vi "Main.vi"(11 "Module Admin":refnum<class "Delacor_lib_QMH_Module Admin.lvclass">) -> ()   [LabVIEW 2022 SP3, in "Settings.lvlib"]
doc: "This template is based off of the Queued Message Handler design pattern and the Queued Message Handler project template that ships with LabVIEW.\n\nThe main difference is that the queue is private to this module and communication between modules is performed via Broadcast and Request events.\n\nRequest events are wrapped in public API methods and are handled in the Event Handling Loop (EHL) of this VI. Any module can register for Broadcast events sent by this module. The EHL generates messages based on user interface actions.\n\nThe Message Handling Loop (MHL) processes messages generated by the EHL, or by other messages. The messages are string values, so new messages can be added easily to the Message Cases case structure in the MHL. Each message cluster can also provide an optional value for Message Data, which is a variant that can be converted to whatever message-specific data is required.\n_____\nBased on DQMH Project Template 7.0.0.1280."
uses:
  Settings.lvlib
  <vilib>/Delacor/Delacor QMH/Libraries/Module Admin_class/Delacor_lib_QMH_Module Admin.lvclass
  Module Data--cluster.ctl
  Do Something Argument--cluster.ctl
  <vilib>/Delacor/Delacor QMH/Libraries/Message Queue_class/Delacor_lib_QMH_Message Queue.lvclass/Delacor_lib_QMH_Message Queue.ctl
  Do Something Else Argument--cluster.ctl
  Do Something Else and Wait for Reply Argument--cluster.ctl
  Do Something Else and Wait (Reply Payload)--cluster.ctl
  Stop Argument--cluster.ctl
  <vilib>/Delacor/Delacor QMH/Libraries/Module Admin_class/Delacor_lib_QMH_Module Admin.lvclass/Delacor_lib_QMH_Module Admin.ctl
  Prepare Argument--cluster.ctl
  Configure Argument--cluster.ctl
  Request UI Display Argument--cluster.ctl
  Framework/UI Manager/Module Display Scenarios.ctl
  Request UI Display (Reply Payload)--cluster.ctl
  <vilib>/Utility/miscctls.llb/LVPointTypeDef.ctl
  <vilib>/Delacor/Delacor QMH/Libraries/Message Queue_class/Delacor_lib_QMH_Enqueue Message (Single).vi
  <vilib>/Delacor/Delacor QMH/Libraries/Module Admin_class/Delacor_lib_QMH_Get External Launch.vi
  <vilib>/Delacor/Delacor QMH/Libraries/Message Queue_class/Delacor_lib_QMH_Message Queue.lvclass
  Libraries/hse-libraries/Source/hse-configuration/config-ini/config-ini.lvclass
  Framework/UI Manager/UI Manager.lvlib
  <vilib>/Hampel Software Engineering/HSE Logger/hse-logger.lvlib
  Libraries/hse-libraries/Source/hse-dqmh/hse-dqmh.lvlib
panel:
  out "error out":errorcluster
  out "X":dbl
  out "Status":string
  in  "Simulate MHL Error":bool
  in  "Simulate EHL Error":bool
  in  "Do Something Else <Replace Me>":bool
  in  "Do Something <Replace Me>":bool
  # "This panel will contain the following configuration settings:\n\n- CAN message build.\n- Neural Network settings.\n- Add user for Facial Recognition."
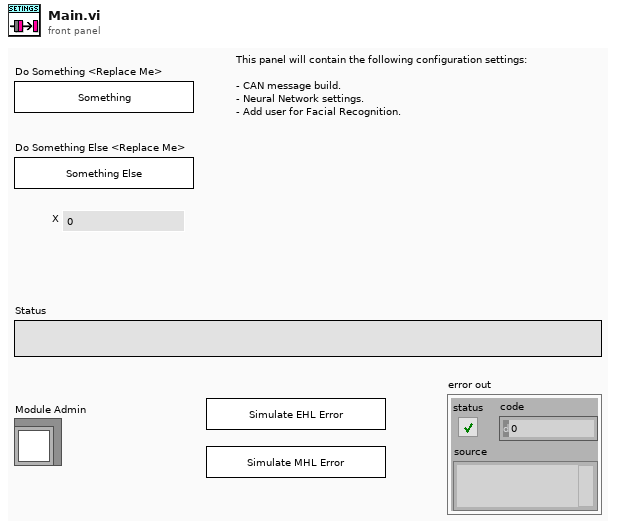
[diagram p1: front panel]
types:
  T1 = typedef "Settings.lvlib/Request Events--cluster.ctl" = cluster{"Stop Module":refnum<user-event>, "Do Something":refnum<user-event>, "Do Something Else":refnum<user-event>, "Do Something Else and Wait for Reply":refnum<user-event>, "Show Panel":refnum<user-event>, "Hide Panel":refnum<user-event>, "Get Module Execution Status":refnum<user-event>, "Show Diagram":refnum<user-event>, "Prepare":refnum<user-event>, "Configure":refnum<user-event>, "Request UI Display":refnum<user-event>}
  T2 = typedef "Settings.lvlib/Module Data--cluster.ctl" = cluster{"Status":string}
  T3 = typedef "Settings.lvlib/Do Something Argument--cluster.ctl" = cluster{"Do Something Msg":string}
  T4 = typedef "Settings.lvlib/Do Something Else Argument--cluster.ctl" = cluster{"Do Something Else Msg":string, "X":dbl}
  T5 = typedef "Settings.lvlib/Do Something Else and Wait for Reply Argument--cluster.ctl" = cluster{"Do Something Else Msg":string, "X":dbl, "Wait Notifier":refnum<notifier>, "wait for reply":bool}
  T6 = enum32{"invalid lock state", "Not Locked", "Locked (No Password)", "Password-protected"}
  T7 = typedef "Settings.lvlib/Stop Argument--cluster.ctl" = cluster{"Origin":string, "Exit via Stop Module Req?":bool, "Wait for Module to stop?":bool}
  T8 = typedef "Settings.lvlib/Prepare Argument--cluster.ctl" = cluster{"Boolean":bool}
  T9 = typedef "Settings.lvlib/Configure Argument--cluster.ctl" = cluster{"Boolean":bool}
  T10 = typedef "Settings.lvlib/Request UI Display Argument--cluster.ctl" = cluster{"Scenario":T11, "Wait Notifier":refnum<notifier>, "wait for reply":bool}
  T11 = typedef "UI Manager.lvlib/Module Display Scenarios.ctl" = enum16{"Stand-Alone", "Managed"}
  T12 = typedef "LVPointTypeDef.ctl" = cluster{"Horizontal":i16, "Vertical":i16}
  T13 = enum32{"Invalid", "Standard", "Closed", "Hidden", "Minimized", "Maximized"}
  T14 = typedef "Settings.lvlib/Do Something Else and Wait (Reply Payload)--cluster.ctl" = cluster{"Value":dbl, "error":errorcluster}
  T15 = typedef "Settings.lvlib/Request UI Display (Reply Payload)--cluster.ctl" = cluster{"Accept":bool, "error":errorcluster}
  T16 = typedef "hse-dqmh.lvlib/System Message Source.ctl" = enum16{"module", "application", "network"}
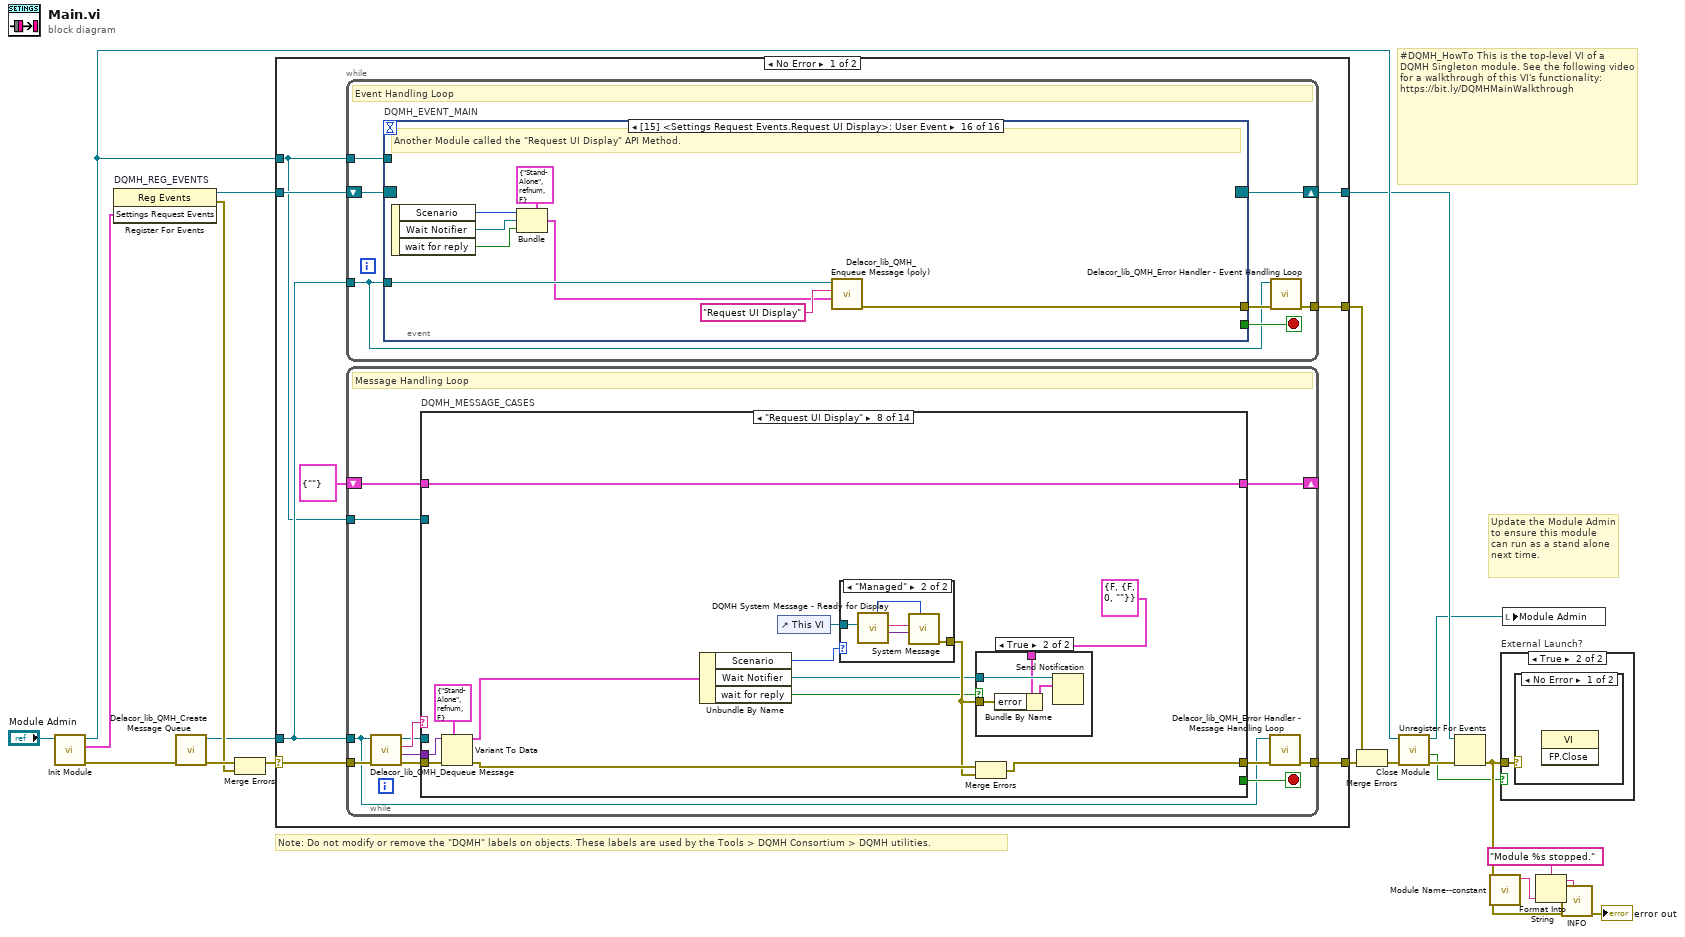
[diagram p0: block diagram]
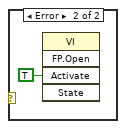
[diagram p3: hidden frame]
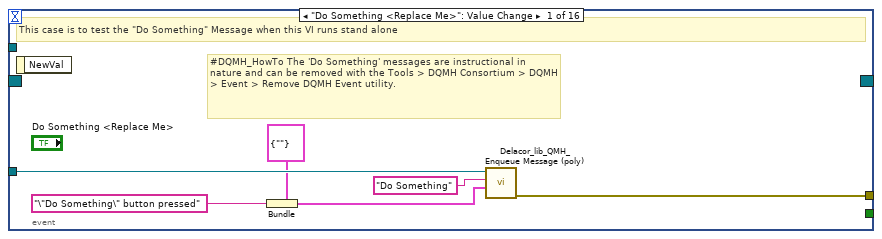
[diagram p4: hidden frame]
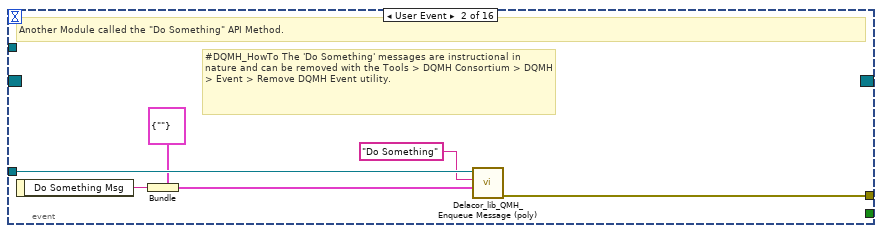
[diagram p5: hidden frame]
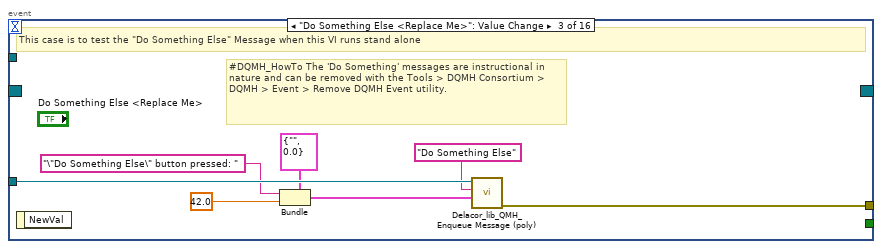
[diagram p6: hidden frame]
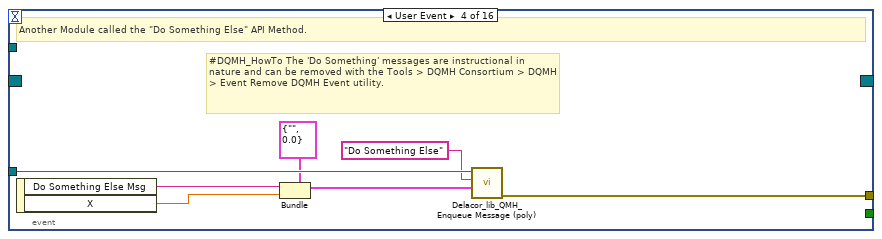
[diagram p7: hidden frame]
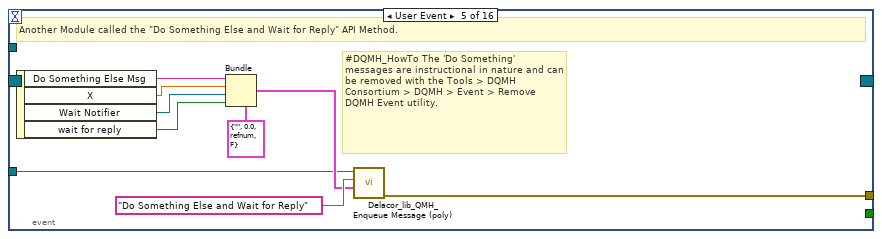
[diagram p8: hidden frame]
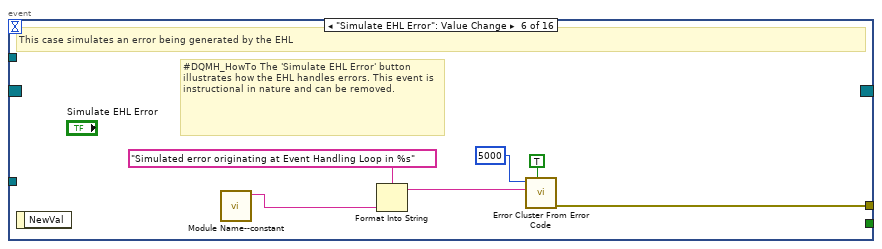
[diagram p9: hidden frame]
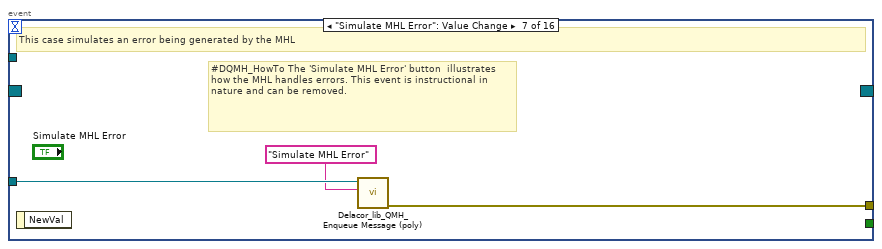
[diagram p10: hidden frame]
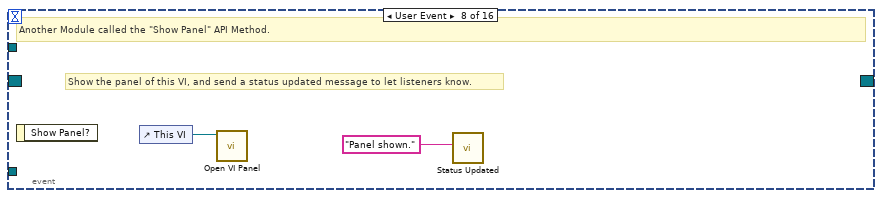
[diagram p11: hidden frame]
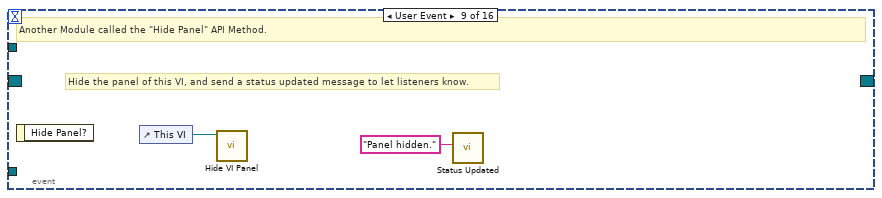
[diagram p12: hidden frame]
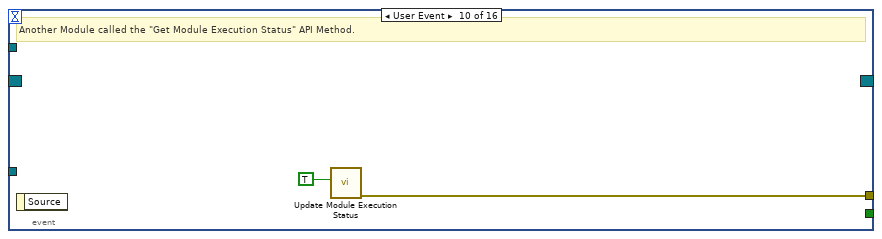
[diagram p13: hidden frame]
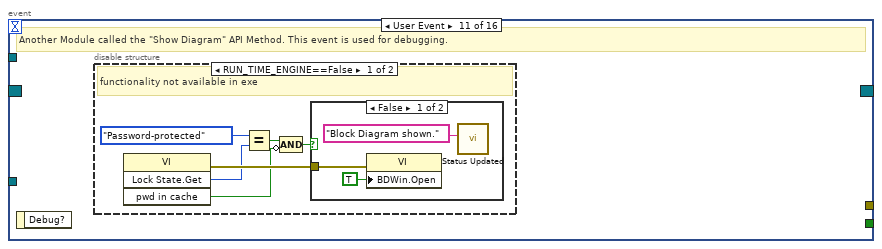
[diagram p14: hidden frame]
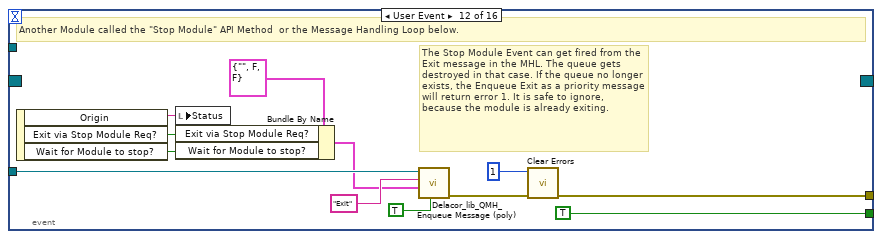
[diagram p17: hidden frame]
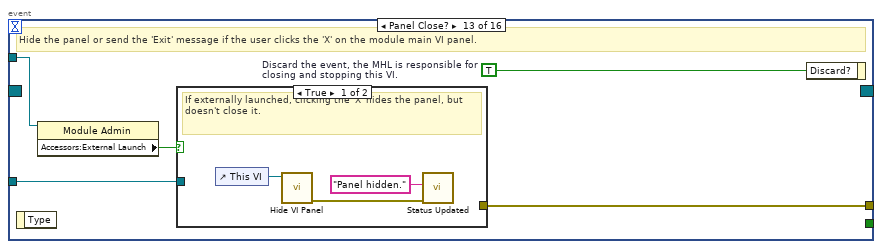
[diagram p18: hidden frame]
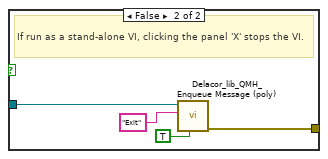
[diagram p19: hidden frame]
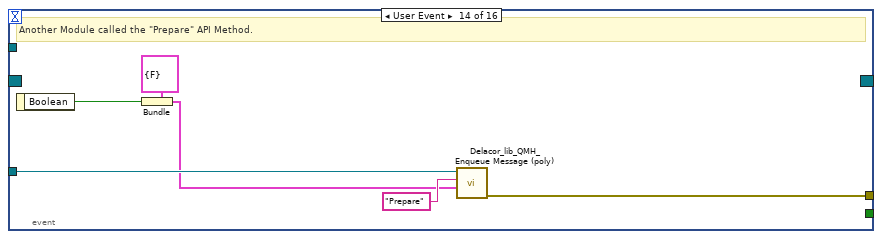
[diagram p20: hidden frame]
diagram:
  # "#DQMH_HowTo This is the top-level VI of a DQMH Singleton module. See the following video for a walkthrough of this VI's functionality: https://bit.ly/DQMHMainWalkthrough"
  # "Note: Do not modify or remove the \"DQMH\" labels on objects. These labels are used by the Tools > DQMH Consortium > DQMH utilities."
  # "Update the Module Admin to ensure this module can run as a stand alone next time."
  n1 = call "Init Module.vi"("Singleton Module Admin in"="Module Admin") -> ("error out"=w20:errorcluster, "Settings Request Events"=w9:T1, "Singleton Module Admin out"=w12:refnum<class "Delacor_lib_QMH_Module Admin.lvclass">)  [unwired: 8 in]
  n2 = register-events "DQMH_REG_EVENTS"(w9) -> (reference out=w10:refnum<event-registration>, error out=w13:errorcluster)  [unwired: 2 in]
  n3 = call <vilib>:"Delacor_lib_QMH_Create Message Queue.vi"("error in"=w20) -> ("error out"=w15:errorcluster, "Message Queue"=w8:refnum<class "Delacor_lib_QMH_Message Queue.lvclass">)  [unwired: 9 in]
  n4 = Merge Errors(w15, w13) -> (w14:errorcluster)
  n5 = case shown="No Error" w14 {
    selector: w14 -> [w27 w334]
    tunnel: [w29 w333] -> w21
    tunnel: [w26 w332] -> w11
    tunnel: w10 -> [w24 w332]
    tunnel: w8 -> [w23 w327]
    tunnel: [w28 _] -> w18
    tunnel: w12 -> [w22 w328]
    frame No Error {
      n6 = while {
        tunnel: w23 -> [w30]
        shift-right: [w33] -> w26
        shift-left: w24 -> [w34]
        tunnel: [w35] -> w28
        tunnel: w22 -> [w31]
        stop <- w32 stop-if-true
        # "Event Handling Loop"
        n7 = event "DQMH_EVENT_MAIN" shown="[15] <Settings Request Events.Request UI Display>: User Event" {
          selector: w34 -> [_ _ _ _ _ _ _ _ _ _ _ _ _ _ _ _]
          dyn-events: [_ _ _ _ _ _ _ _ _ _ _ _ _ _ _ _] -> w33
          timeout: _ -> [_ _ _ _ _ _ _ _ _ _ _ _ _ _ _ _]
          tunnel: [_ _ _ _ _ _ _ _ _ _ _ TRUE ("Discard?") _ _ _ _] -> w32
          tunnel: w30 -> [w41 w47 w54 w61 w64 _ w79 _ _ _ _ w103 w110 w125 w131 w139]
          tunnel: [w42 w48 w55 w62 w71 w77 w80 _ _ w86 _ w106 w112 w120 w126 w132] -> w36
          tunnel: w31 -> [_ _ _ _ _ _ _ _ _ _ _ _ w109 _ _ _]
          event "Do Something <Replace Me>": Value Change {
            # "#DQMH_HowTo The 'Do Something' messages are instructional in nature and can be removed with the Tools > DQMH Consortium > DQMH > Event > Remove DQMH Event utility."
            # "This case is to test the \"Do Something\" Message when this VI runs stand alone"
            n8 = event-data() -> ()  [unwired: 1 in, 1 out]
            n9 = Bundle(cluster=T3 {"Do Something Msg"=""} ("Do Something Argument"), "Do Something Msg"="\"Do Something\" button pressed" ("\"Do Something\" button pressed")) -> (w37:T3)
            n10 = call-poly <vilib>:"Delacor_lib_QMH_Enqueue Message (poly).vi"("Message Data"=w37, "Message"="Do Something", "Message Queue in"=w41) -> ("error out"=w42:errorcluster)  [unwired: 7 in, 1 out]
          }
          event User Event {
            # "#DQMH_HowTo The 'Do Something' messages are instructional in nature and can be removed with the Tools > DQMH Consortium > DQMH > Event > Remove DQMH Event utility."
            # "Another Module called the \"Do Something\" API Method."
            n11 = event-data() -> ("Do Something Msg"=w44:string)  [unwired: 1 in]
            n12 = Bundle(cluster=T3 {"Do Something Msg"=""} ("Do Something Argument"), "Do Something Msg"=w44) -> (w43:T3)
            n13 = call-poly <vilib>:"Delacor_lib_QMH_Enqueue Message (poly).vi"("Message Data"=w43, "Message"="Do Something", "Message Queue in"=w47) -> ("error out"=w48:errorcluster)  [unwired: 7 in, 1 out]
          }
          event "Do Something Else <Replace Me>": Value Change {
            # "#DQMH_HowTo The 'Do Something' messages are instructional in nature and can be removed with the Tools > DQMH Consortium > DQMH > Event > Remove DQMH Event utility."
            # "This case is to test the \"Do Something Else\" Message when this VI runs stand alone"
            n14 = event-data() -> ()  [unwired: 1 in, 1 out]
            n15 = Bundle(cluster=T4 {"Do Something Else Msg"="", "X"=0.0} ("Do Something Else Argument"), "Do Something Else Msg"="\"Do Something Else\" button pressed: " ("\"Do Something Else\" button pressed"), "X"=42.0) -> (w51:T4)
            n16 = call-poly <vilib>:"Delacor_lib_QMH_Enqueue Message (poly).vi"("Message Data"=w51, "Message"="Do Something Else", "Message Queue in"=w54) -> ("error out"=w55:errorcluster)  [unwired: 7 in, 1 out]
          }
          event User Event {
            # "#DQMH_HowTo The 'Do Something' messages are instructional in nature and can be removed with the Tools > DQMH Consortium > DQMH > Event Remove DQMH Event utility."
            # "Another Module called the \"Do Something Else\" API Method."
            n17 = event-data() -> ("Do Something Else Msg"=w57:string, "X"=w56:dbl)  [unwired: 1 in]
            n18 = Bundle(cluster=T4 {"Do Something Else Msg"="", "X"=0.0} ("Do Something Else Argument"), "Do Something Else Msg"=w57, "X"=w56) -> (w58:T4)
            n19 = call-poly <vilib>:"Delacor_lib_QMH_Enqueue Message (poly).vi"("Message Data"=w58, "Message"="Do Something Else", "Message Queue in"=w61) -> ("error out"=w62:errorcluster)  [unwired: 7 in, 1 out]
          }
          event User Event {
            # "#DQMH_HowTo The 'Do Something' messages are instructional in nature and can be removed with the Tools > DQMH Consortium > DQMH > Event > Remove DQMH Event utility."
            # "Another Module called the \"Do Something Else and Wait for Reply\" API Method."
            n20 = event-data() -> ("Do Something Else Msg"=w67:string, "X"=w66:dbl, "Wait Notifier"=w65:refnum<notifier>, "wait for reply"=w63:bool)  [unwired: 1 in]
            n21 = Bundle(cluster=T5 {"Do Something Else Msg"="", "X"=0.0, "Wait Notifier"=refnum, "wait for reply"=FALSE} ("Do Something Else and Wait for Reply Argument"), "Do Something Else Msg"=w67, "X"=w66, "Wait Notifier"=w65, "wait for reply"=w63) -> (w68:T5)
            n22 = call-poly <vilib>:"Delacor_lib_QMH_Enqueue Message (poly).vi"("Message Data"=w68, "Message"="Do Something Else and Wait for Reply", "Message Queue in"=w64) -> ("error out"=w71:errorcluster)  [unwired: 7 in, 1 out]
          }
          event "Simulate EHL Error": Value Change {
            # "#DQMH_HowTo The 'Simulate EHL Error' button  illustrates how the EHL handles errors. This event is instructional in nature and can be removed."
            # "This case simulates an error being generated by the EHL"
            n23 = event-data() -> ()  [unwired: 1 in, 1 out]
            n24 = call "Module Name--constant.vi"() -> ("Module Name"=w74:string)  [unwired: 11 in]
            n25 = Format Into String(format string="Simulated error originating at Event Handling Loop in %s", w74) -> (resulting string=w75:string)  [unwired: 2 in, 1 out]
            n26 = call <vilib>:"Error Cluster From Error Code.vi"("show call chain? (False)"=TRUE, "error message (\"\")"=w75, "error code (0)"=5000) -> ("error out"=w77:errorcluster)  [unwired: 6 in]
          }
          event "Simulate MHL Error": Value Change {
            # "#DQMH_HowTo The 'Simulate MHL Error' button  illustrates how the MHL handles errors. This event is instructional in nature and can be removed."
            # "This case simulates an error being generated by the MHL"
            n27 = event-data() -> ()  [unwired: 1 in, 1 out]
            n28 = call-poly <vilib>:"Delacor_lib_QMH_Enqueue Message (poly).vi"("Message"="Simulate MHL Error", "Message Queue in"=w79) -> ("error out"=w80:errorcluster)  [unwired: 8 in, 1 out]
          }
          event User Event {
            # "Show the panel of this VI, and send a status updated message to let listeners know."
            # "Another Module called the \"Show Panel\" API Method."
            n29 = event-data() -> ()  [unwired: 1 in, 1 out]
            n30 = control-ref of="This VI"() -> (w82:refnum<vi>)
            n31 = call "Open VI Panel.vi"("VI"=w82) -> ()  [unwired: 10 in, 1 out]
            n32 = call "Status Updated.vi"("Status"="Panel shown." ("format string")) -> ()  [unwired: 10 in, 1 out]
          }
          event User Event {
            # "Hide the panel of this VI, and send a status updated message to let listeners know."
            # "Another Module called the \"Hide Panel\" API Method."
            n33 = event-data() -> ()  [unwired: 1 in, 1 out]
            n34 = control-ref of="This VI"() -> (w84:refnum<vi>)
            n35 = call "Hide VI Panel.vi"("VI"=w84) -> ()  [unwired: 10 in, 1 out]
            n36 = call "Status Updated.vi"("Status"="Panel hidden." ("format string")) -> ()  [unwired: 10 in, 1 out]
          }
          event User Event {
            # "Another Module called the \"Get Module Execution Status\" API Method."
            n37 = event-data() -> ()  [unwired: 1 in, 1 out]
            n38 = call "Update Module Execution Status.vi"("Running?"=TRUE) -> ("error out"=w86:errorcluster)  [unwired: 10 in]
          }
          event User Event {
            # "Another Module called the \"Show Diagram\" API Method. This event is used for debugging."
            n39 = event-data() -> ()  [unwired: 1 in, 1 out]
            n40 = disable-structure shown="RUN_TIME_ENGINE==False" {
              frame condition #0 (active) {
                # "functionality not available in exe"
                n41 = invoke class="VI" method="Lock State.Get"() -> (error out=w92:errorcluster, "Get Lock State"=w91:T6, "pwd in cache"=w88:bool)  [unwired: 4 in, 1 out]
                n42 = Equal?(x=T6."Password-protected", y=w91) -> (x = y?=w89:bool)
                n43 = Compound Arithmetic op=AND(w89, invert w88) -> (w87:bool)
                n44 = case shown="False" w87 {
                  tunnel: w92 -> [w95 _]
                  frame False {
                    n45 = property class="VI"(error in=w95, "BDWin.Open"=TRUE ("Block Diagram Window:Open")) -> ()  [unwired: 1 in, 2 out]
                    n46 = call "Status Updated.vi"("Status"="Block Diagram shown." ("format string")) -> ()  [unwired: 10 in, 1 out]
                  }
                  frame True {
                    # "Password-protected VI, and the password is not in the cache. Do not show the diagram."
                  }
                }
              }
              frame condition #1 {
              }
            }
          }
          event User Event {
            # "The Stop Module Event can get fired from the Exit message in the MHL. The queue gets destroyed in that case. If the queue no longer exists, the Enqueue Exit as a priority message will return error 1. It is safe to ignore, because the module is already exiting."
            # "Another Module called the \"Stop Module\" API Method  or the Message Handling Loop below."
            n47 = event-data() -> ("Origin"=w102:string, "Exit via Stop Module Req?"=w98:bool, "Wait for Module to stop?"=w97:bool)  [unwired: 1 in]
            n48 = local write "Status"(w102) -> ()
            n49 = Bundle By Name(cluster=T7 {"Origin"="", "Exit via Stop Module Req?"=FALSE, "Wait for Module to stop?"=FALSE} ("Stop Argument"), "Exit via Stop Module Req?"=w98, "Wait for Module to stop?"=w97) -> (w96:T7)
            n50 = call-poly <vilib>:"Delacor_lib_QMH_Enqueue Message (poly).vi"("Priority Message? (F)"=TRUE, "Message Data"=w96, "Message"="Exit", "Message Queue in"=w103) -> ("error out"=w107:errorcluster)  [unwired: 6 in, 1 out]
            n51 = call <vilib>:"Clear Errors.vi"("error in (no error)"=w107, "specific error code to clear (0: all)"=1) -> ("error out"=w106:errorcluster)  [unwired: 4 in, 1 out]
          }
          event Panel Close? {
            w111 = TRUE  # Discard the event, the MHL is responsible for closing and stopping this VI.
            # "Hide the panel or send the 'Exit' message if the user clicks the 'X' on the module main VI panel."
            n52 = event-data() -> ()  [unwired: 1 in, 1 out]
            n53 = property class="Module Admin"(reference=w109) -> ("Accessors:External Launch"=w108:bool)  [unwired: 1 in, 2 out]
            n54 = case shown="True" w108 {
              tunnel: w110 -> [_ w118]
              tunnel: [_ w119] -> w112
              frame True {
                # "If externally launched, clicking the 'X' hides the panel, but doesn't close it."
                n55 = control-ref of="This VI"() -> (w115:refnum<vi>)
                n56 = call "Hide VI Panel.vi"("VI"=w115) -> ("error out"=w113:errorcluster)  [unwired: 10 in]
                n57 = call "Status Updated.vi"("error in"=w113, "Status"="Panel hidden." ("format string")) -> ()  [unwired: 9 in, 1 out]
              }
              frame False {
                # "If run as a stand-alone VI, clicking the panel 'X' stops the VI."
                n58 = call-poly <vilib>:"Delacor_lib_QMH_Enqueue Message (poly).vi"("Priority Message? (F)"=TRUE, "Message"="Exit", "Message Queue in"=w118) -> ("error out"=w119:errorcluster)  [unwired: 7 in, 1 out]
              }
            }
            n59 = event-data("Discard?"=w111) -> ()  [unwired: 1 in, 1 out]
          }
          event User Event {
            # "Another Module called the \"Prepare\" API Method."
            n60 = event-data() -> ("Boolean"=w121:bool)  [unwired: 1 in]
            n61 = Bundle(cluster=T8 {"Boolean"=FALSE} ("Prepare Argument"), "Boolean"=w121) -> (w122:T8)
            n62 = call-poly <vilib>:"Delacor_lib_QMH_Enqueue Message (poly).vi"("Message Data"=w122, "Message"="Prepare", "Message Queue in"=w125) -> ("error out"=w120:errorcluster)  [unwired: 7 in, 1 out]
          }
          event User Event {
            # "Another Module called the \"Configure\" API Method."
            n63 = event-data() -> ("Boolean"=w127:bool)  [unwired: 1 in]
            n64 = Bundle(cluster=T9 {"Boolean"=FALSE} ("Configure Argument"), "Boolean"=w127) -> (w128:T9)
            n65 = call-poly <vilib>:"Delacor_lib_QMH_Enqueue Message (poly).vi"("Message Data"=w128, "Message"="Configure", "Message Queue in"=w131) -> ("error out"=w126:errorcluster)  [unwired: 7 in, 1 out]
          }
          event User Event {
            # "Another Module called the \"Request UI Display\" API Method."
            n66 = event-data() -> ("Scenario"=w135:T11, "Wait Notifier"=w134:refnum<notifier>, "wait for reply"=w133:bool)  [unwired: 1 in]
            n67 = Bundle(cluster=T10 {"Scenario"=enum."Stand-Alone", "Wait Notifier"=refnum, "wait for reply"=FALSE} ("Request UI Display Argument"), "Scenario"=w135, "Wait Notifier"=w134, "wait for reply"=w133) -> (w136:T10)
            n68 = call-poly <vilib>:"Delacor_lib_QMH_Enqueue Message (poly).vi"("Message Data"=w136, "Message"="Request UI Display", "Message Queue in"=w139) -> ("error out"=w132:errorcluster)  [unwired: 7 in, 1 out]
          }
        }
        n69 = call-dynamic "Delacor_lib_QMH_Error Handler - Event Handling Loop.vi"("error in"=w36, "Message Queue in"=w30) -> ("dup error in"=w35:errorcluster)  [unwired: 8 in, 1 out]
      }
      n70 = while {
        tunnel: w23 -> [w140]
        shift-right: [w146] -> _
        shift-left: T2 {"Status"=""} ("Data Cluster") -> [w147]
        tunnel: w27 -> [w150]
        tunnel: [w148] -> w29
        tunnel: w22 -> [w141]
        stop <- w145 stop-if-true
        # "Message Handling Loop"
        n71 = call-dynamic "Delacor_lib_QMH_Dequeue Message.vi"("error in"=w150, "Message Queue in"=w140) -> ("error out"=w149:errorcluster, "Message Data"=w143:variant, "Message"=w144:string, "Message Queue out"=w142:refnum<class "Delacor_lib_QMH_Message Queue.lvclass">)  [unwired: 6 in]
        n72 = case "DQMH_MESSAGE_CASES" shown="\"Request UI Display\"" w144 {
          selector: w144 -> [_ _ _ _ _ _ _ _ _ _ _ _ _ w322]
          tunnel: w142 -> [_ _ _ _ _ _ _ _ _ _ _ w288 w310 _]
          tunnel: w149 -> [w172 w176 w184 w193 w212 w228 w243 w257 w271 w273 w282 w295 w316 w325]
          tunnel: [w154 w176 w182 w192 w211 w226 w242 w252 w270 w273 w281 w291 w311 w326] -> w151
          tunnel: w147 -> [w161 w175 w181 w191 w208 w227 w244 w256 w269 w272 w279 w290 w309 w323]
          tunnel: [w160 w175 w181 w191 w208 w227 w244 w256 w269 w272 w279 w290 w309 w323] -> w146
          tunnel: [_ _ _ _ _ _ _ _ _ _ _ _ w308 _] -> w145
          tunnel: w143 -> [_ _ w180 w188 w205 w225 _ w254 _ _ _ w289 w307 _]
          tunnel: w141 -> [w162 _ _ _ _ _ _ _ _ _ _ w287 w302 _]
          frame "Initialize" {
            w156 = "Initial Message" ("Initial Message")
            # "#CodeNeeded - Initialize the appearance of the front panel."
            # "#CodeNeeded - Initialize your state data here."
            # "Initialize - Any operation that needs to be done before the module can receive messages. Synchronize Caller Events.vi will inform Start Module.vi that the module has launched and is ready to receive messages. Module Did Init.vi will broadcast that the module initialized."
            n73 = call "Synchronize Caller Events.vi"("error in"=w172, "Singleton Module Admin in"=w162) -> ("error out"=w171:errorcluster, "Singleton Module Admin out"=w157:refnum<class "Delacor_lib_QMH_Module Admin.lvclass">)  [unwired: 8 in]
            n74 = property class="Module Admin"(reference=w157) -> ("Accessors:External Launch"=w166:bool)  [unwired: 1 in, 2 out]
            n75 = Select(t=T13."Hidden" ("State"), s=w166, f=T13."Standard" ("State")) -> (s? t:f=w163:T13)
            n76 = call "Module Name--constant.vi"() -> ("Module Name"=w158:string)  [unwired: 11 in]
            n77 = call "Module Name--constant.vi"() -> ("Module Name"=w169:string)  [unwired: 11 in]
            n78 = property class="VI"("Front Panel.Title"=w169) -> (reference out=w168:refnum<vi>, error out=w174:errorcluster)  [unwired: 2 in]
            n79 = call "Module Did Init.vi"("error in"=w171, "Initialized?"=TRUE, "Origin"=w158) -> ("error out"=w170:errorcluster)  [unwired: 8 in]
            n80 = invoke class="VI" method="FP.Open"(reference=w168, error in=w174, "State"=w163) -> (reference out=w167:refnum<vi>, error out=w173:errorcluster)  [unwired: 2 in, 3 out]
            n81 = Bundle By Name(cluster=w161, "Status"=w156) -> (w160:T2)
            n82 = invoke class="VI" method="FP.Center"(reference=w167, error in=w173) -> ()  [unwired: 1 in, 3 out]
            n83 = property on="Pane" class="Pane"("Origin"=T12 {"Horizontal"=0, "Vertical"=0}) -> ()  [unwired: 2 in, 2 out]
            n84 = Format Into String(format string="Module %s started.", w158) -> (resulting string=w152:string)  [unwired: 2 in, 1 out]
            n85 = call <vilib>:"INFO.vi"("Message"=w152, "error in"=w170) -> ("error out"=w154:errorcluster)  [unwired: 9 in]
            "Status" <- w156
          }
          frame "---Module Specific---" {
            # "Separator -- The following cases handle messages specific to this Module."
          }
          frame "Do Something" {
            # "#DQMH_HowTo The 'Do Something' messages are instructional in nature and can be removed with the Tools > DQMH Consortium > DQMH > Event > Remove DQMH Event utility."
            # "Do Something - Replace this message with functionality for your own application. Note that this message also fires the \"Did Something\" broadcast event."
            n86 = Variant To Data(error in=w184, type=T3 {"Do Something Msg"=""} ("Do Something Argument"), Variant=w180) -> (data=w179:T3, error out=w183:errorcluster)
            n87 = Unbundle By Name(w179) -> ("Do Something Msg"=w177:string)
            n88 = call "Did Something.vi"("error in"=w183, "Did Something Msg"=w177) -> ("error out"=w182:errorcluster)  [unwired: 9 in]
            n89 = local write "Status"(w177) -> ()
            n90 = call "Status Updated.vi"("Status"=w177) -> ()  [unwired: 10 in, 1 out]
          }
          frame "Do Something Else" {
            # "#DQMH_HowTo The 'Do Something' messages are instructional in nature and can be removed with the Tools > DQMH Consortium > DQMH > Event > Remove DQMH Event utility."
            # "Do Something Else - Replace this message with functionality for your own application."
            n91 = Variant To Data(error in=w193, type=T4 {"Do Something Else Msg"="", "X"=0.0} ("Do Something Else Argument"), Variant=w188) -> (data=w189:T4, error out=w192:errorcluster)
            n92 = Unbundle By Name(w189) -> ("Do Something Else Msg"=w187:string, "X"=w186:dbl)
            "X" <- w186
            n93 = Format Into String(initial string=w187, w186) -> (resulting string=w185:string)  [unwired: 2 in, 1 out]
            n94 = local write "Status"(w185) -> ()
            n95 = call "Status Updated.vi"("Status"=w185) -> ()  [unwired: 10 in, 1 out]
          }
          frame "Do Something Else and Wait for Reply" {
            w200 = "X(%.2f)+Offset(%.2f)=%.2f"  # status message format string
            # "#DQMH_HowTo The 'Do Something' messages are instructional in nature and can be removed."
            # "Send back X with a random offset"
            # "Do Something Else and Wait for Reply - Replace this message with functionality for your own application. Note that this message must fire a notifier to let callers know it has finished execution, and it returns an error if the 'Value' is negative."
            n96 = Variant To Data(error in=w212, type=T5 {"Do Something Else Msg"="", "X"=0.0, "Wait Notifier"=refnum, "wait for reply"=FALSE} ("Do Something Else and Wait for Reply Argument"), Variant=w205) -> (data=w206:T5, error out=w210:errorcluster)
            n97 = Unbundle By Name(w206) -> ("Wait Notifier"=w194:refnum<notifier>, "Do Something Else Msg"=w204:string, "X"=w201:dbl, "wait for reply"=w197:bool)
            n98 = Random Number (0-1)() -> (number: 0 to 1=w202:dbl)
            n99 = Add(x=w202, y=w201) -> (x+y=w196:dbl)
            n100 = Less Than 0?(x=w196) -> (x < 0?=w199:bool)
            n101 = local write "X"(w201) -> ()
            n102 = case shown="True" w199 {
              tunnel: [_ w222] -> w209
              frame False {
              }
              frame True {
                n103 = call <vilib>:"Error Cluster From Error Code.vi"("show call chain? (False)"=TRUE, "error message (\"\")"="The 'Something Else and Wait for Reply' message generated a negative number, which is considered an error condition.", "error code (0)"=5000) -> ("error out"=w222:errorcluster)  [unwired: 6 in]
              }
            }
            n104 = Format Into String(format string=w200, initial string=w204, w201, w202, w196) -> (resulting string=w198:string)  [unwired: 1 in, 1 out]
            n105 = Bundle By Name(cluster=T14 {"Value"=0.0, "error"={"status"=FALSE, "code"=0, "source"=""}} ("notification"), "error"=w209, "Value"=w196) -> (w195:T14)
            n106 = local write "Status"(w198) -> ()
            n107 = call "Status Updated.vi"("Status"=w198) -> ()  [unwired: 10 in, 1 out]
            n108 = case shown="True" w197 {
              tunnel: w195 -> [_ w215]
              tunnel: w194 -> [_ w214]
              frame False {
              }
              frame True {
                # "Simulate an operation that requires a wait."
                n109 = flat-sequence {
                  tunnel: w215 -> [w218]
                  tunnel: w214 -> [w217]
                  tunnel: w213 -> [_]
                  frame #0 {
                    n110 = Send Notification(notification=w218, notifier=w217) -> ()  [unwired: 1 in, 2 out]
                  }
                }
                n111 = Wait (ms)(milliseconds to wait=u32 1000) -> (millisecond timer value=w213:u32)
              }
            }
            n112 = Merge Errors(w210, w209) -> (w211:errorcluster)
          }
          frame "Prepare" {
            # "#CodeNeeded\n1. Configure this Message Case for handling the \"Prepare\" message.\n2. Delete or edit this label when done."
            n113 = Variant To Data(error in=w228, type=T8 {"Boolean"=FALSE} ("Prepare Argument"), Variant=w225) -> (data=w223:T8, error out=w226:errorcluster)
            n114 = Unbundle By Name(w223) -> ()  [unwired: 1 out]
          }
          frame "Configure" {
            n115 = call "Module Name--constant.vi"() -> ("Module Name"=w237:string)  [unwired: 11 in]
            n116 = call "Create Module Config.vi"("error in"=w243, "DQMH Module Name"=w237) -> ("error out"=w239:errorcluster, "config-ini out"=w238:refnum<class "config-ini.lvclass">)  [unwired: 8 in]
            n117 = control-ref of="This VI"() -> (w230:refnum<vi>)
            n118 = call-dynamic "Read String.vi"("Section"="global" ("global"), "error in"=w239, "Key"="descriptor" ("descriptor"), "config-base in"=w238) -> ("error out"=w234:errorcluster, "Value"=w229:string)  [unwired: 5 in, 1 out]
            n119 = property class="VI"(reference=w230, "Front Panel.Title"=w229) -> ()  [unwired: 1 in, 2 out]
            n120 = call "DQMH System Message - Add to Run-Time Menu.vi"("Module Descriptor"=w229, "Main VI Reference"=w230) -> ("Payload"=w231:variant, "Identifier"=w232:string, "Source"=w233:T16)  [unwired: 7 in]
            n121 = Format Into String(format string="Module %s configured.", w237) -> (resulting string=w235:string)  [unwired: 2 in, 1 out]
            n122 = call "System Message.vi"("Sys. Msg. Source"=w233, "Payload"=w231, "Identifier"=w232) -> ()  [unwired: 8 in, 1 out]
            n123 = call <vilib>:"INFO.vi"("Message"=w235, "error in"=w234) -> ("error out"=w242:errorcluster)  [unwired: 9 in]
          }
          frame "Request UI Display" {
            n124 = Variant To Data(error in=w257, type=T10 {"Scenario"=enum."Stand-Alone", "Wait Notifier"=refnum, "wait for reply"=FALSE} ("Request UI Display Argument"), Variant=w254) -> (data=w250:T10, error out=w255:errorcluster)
            n125 = Unbundle By Name(w250) -> ("Scenario"=w247:T11, "Wait Notifier"=w245:refnum<notifier>, "wait for reply"=w246:bool)
            n126 = control-ref of="This VI"() -> (w248:refnum<vi>)
            n127 = case shown="\"Managed\"" w247 {
              tunnel: w248 -> [w259 w260]
              tunnel: [w258 w261] -> w249
              frame "Stand-Alone", Default {
                n128 = call "Open VI Panel.vi"("VI"=w259) -> ("error out"=w258:errorcluster)  [unwired: 10 in]
              }
              frame "Managed" {
                n129 = call "DQMH System Message - Ready for Display.vi"("Main VI Reference"=w260) -> ("Payload"=w264:variant, "Identifier"=w263:string, "Source"=w262:T16)  [unwired: 8 in]
                n130 = call "System Message.vi"("Sys. Msg. Source"=w262, "Payload"=w264, "Identifier"=w263) -> ("error out"=w261:errorcluster)  [unwired: 8 in]
              }
            }
            n131 = case shown="True" w246 {
              tunnel: w245 -> [_ w268]
              tunnel: T15 {"Accept"=FALSE, "error"={"status"=FALSE, "code"=0, "source"=""}} ("Request UI Display (Reply Payload)") -> [_ w267]
              tunnel: w249 -> [_ w265]
              frame False {
              }
              frame True {
                n132 = Bundle By Name(cluster=w267, "error"=w265) -> (w266:T15)
                n133 = Send Notification(notification=w266, notifier=w268) -> ()  [unwired: 1 in, 2 out]
              }
            }
            n134 = Merge Errors(w255, w249) -> (w252:errorcluster)
          }
          frame "---Copy This Frame---" {
            # "Duplicate this frame when creating new messages.  Change this comment in the duplicated frame to describe this message."
            n135 = Merge Errors(w271) -> (w270:errorcluster)
          }
          frame "---Exit and Error Handling---" {
            # "Separator - The following cases handle errors and exit messages."
          }
          frame "Simulate MHL Error" {
            # "#DQMH_HowTo The 'Simulate MHL Error' button  illustrates how the MHL handles errors. This event is instructional in nature and can be removed."
            # "Simulate an error occurring at the MHL"
            n136 = call "Module Name--constant.vi"() -> ("Module Name"=w275:string)  [unwired: 11 in]
            n137 = Format Into String(format string="Simulated error originating at Message Handling Loop in %s", w275) -> (resulting string=w276:string)  [unwired: 2 in, 1 out]
            n138 = call <vilib>:"Error Cluster From Error Code.vi"("show call chain? (False)"=TRUE, "error message (\"\")"=w276, "error code (0)"=5001) -> ("error out"=w280:errorcluster)  [unwired: 6 in]
            n139 = Merge Errors(w282, w280) -> (w281:errorcluster)
          }
          frame "Error" {
            # "#CodeRecommended - If the module is running in standalone mode (External Launch = FALSE), this code will pop up an error dialog and call the 'Exit' message if an error occurs. Add more fine-grained error management here."
            # "Error - Check the error message data and respond accordingly. This message is sent by the \"Error Handler\" VIs at the end of each loop in this application."
            n140 = property class="Module Admin"(reference=w287) -> ("Accessors:External Launch"=w286:bool)  [unwired: 1 in, 2 out]
            n141 = Variant To Data(error in=w295, type=errorcluster {"status"=FALSE, "code"=0, "source"=""} ("error constant"), Variant=w289) -> (data=w285:errorcluster, error out=w293:errorcluster)
            n142 = local write "error out"(w285) -> ()
            n143 = call <vilib>:"ERROR.vi"("Message"="DQMH Error Case", "error in"=w285) -> ("error out"=w284:errorcluster)  [unwired: 9 in]
            n144 = call "Error Reported.vi"("Error"=w285) -> ()  [unwired: 10 in, 1 out]
            n145 = case shown="False" w286 {
              tunnel: [w300 _] -> w292
              tunnel: w288 -> [w298 _]
              tunnel: w284 -> [w299 _]
              frame False {
                n146 = disable-structure shown="Default" {
                  disable-tunnel: w299 -> [w301 _]
                  frame condition #0 (active) {
                    # "If the module is running standalone, then pop up an error dialog and call the \"Exit\" message."
                    n147 = call <vilib>:"Simple Error Handler.vi"("error in (no error)"=w301) -> ()  [unwired: 4 in, 5 out]
                  }
                  frame condition #1 {
                    # "To prevent the Simple Error Handler VI from being loaded (e.g. when deploying to a Real-Time target), add the Conditional Disable Symbol \"DQMH_Disable_SEH\" to your project and set it to TRUE."
                  }
                }
                n148 = call-poly <vilib>:"Delacor_lib_QMH_Enqueue Message (poly).vi"("Priority Message? (F)"=TRUE, "Message"="Exit", "Message Queue in"=w298) -> ("error out"=w300:errorcluster)  [unwired: 7 in, 1 out]
              }
              frame True {
                # "If the module was launched externally, calling the Error Reported broadcast VI is the only action performed by the \"Error\" message. The module's caller can then process the error appropriately."
              }
            }
            n149 = Merge Errors(w293, w292) -> (w291:errorcluster)
          }
          frame "Exit" {
            w306 = 91  # 91: not all Exit messages will have an argument
            w308 = TRUE  # Stop the VI
            # "Release the message queue reference"
            # "#CodeNeeded - Add any required cleanup code here."
            # "Exit - Exit the application."
            n150 = Variant To Data(error in=w316, type=T7 {"Origin"="", "Exit via Stop Module Req?"=FALSE, "Wait for Module to stop?"=FALSE} ("Stop Argument"), Variant=w307) -> (data=w304:T7, error out=w313:errorcluster)
            n151 = call <vilib>:"Clear Errors.vi"("error in (no error)"=w313, "specific error code to clear (0: all)"=w306) -> ("error out"=w315:errorcluster)  [unwired: 4 in, 1 out]
            n152 = control-ref of="This VI"() -> (w303:refnum<vi>)
            n153 = call-dynamic "Delacor_lib_QMH_Release Message Queue.vi"("error in"=w315, "Message Queue"=w310) -> ("error out"=w314:errorcluster)  [unwired: 9 in]
            n154 = call "Handle Exit.vi"("Stop Argument"=w304, "Admin in"=w302, "VI reference"=w303) -> ("error out"=w312:errorcluster)  [unwired: 7 in, 1 out]
            n155 = Merge Errors(w314, w312) -> (w311:errorcluster)
            n156 = call "Error Reported.vi"("Error"=w311) -> ()  [unwired: 10 in, 1 out]
          }
          frame Default {
            # "'Default' case only runs if there is a message that isn't defined in any of the other cases.  Output a programming error."
            n157 = call "Module Name--constant.vi"() -> ("Module Name"=w321:string)  [unwired: 11 in]
            n158 = Format Into String(format string="The invalid message string \"%s\" was received in the Message Handling Loop for module \"%s\".", w322, w321) -> (resulting string=w317:string)  [unwired: 2 in, 1 out]
            n159 = call <vilib>:"Error Cluster From Error Code.vi"("show call chain? (False)"=TRUE, "error message (\"\")"=w317, "error code (0)"=1) -> ("error out"=w324:errorcluster)  [unwired: 6 in]
            n160 = Merge Errors(w325, w324) -> (w326:errorcluster)
          }
        }
        n161 = call-dynamic "Delacor_lib_QMH_Error Handler - Message Handling Loop.vi"("error in"=w151, "Message Queue in"=w140) -> ("dup error in"=w148:errorcluster)  [unwired: 8 in, 1 out]
      }
    }
    frame Error {
      # "Synchronize Caller Events.vi will inform Start Module.vi that the module has launched and will let the code calling Start Module.vi register for broadcasts and would permit the caller receive the broadcast that an error occurred at launch time."
      n162 = call-dynamic "Delacor_lib_QMH_Release Message Queue.vi"("error in"=w334, "Message Queue"=w327) -> ("error out"=w333:errorcluster)  [unwired: 9 in]
      n163 = call "Synchronize Caller Events.vi"("Singleton Module Admin in"=w328) -> ("error out"=w335:errorcluster)  [unwired: 9 in, 1 out]
      n164 = call "Module Name--constant.vi"() -> ("Module Name"=w331:string)  [unwired: 11 in]
      n165 = Format Into String(format string="An error occurred during initialization. %s is no longer running.", w331) -> (resulting string=w329:string)  [unwired: 2 in, 1 out]
      n166 = Merge Errors(w333, w335) -> (w336:errorcluster)
      n167 = call "Error Reported.vi"("Additional Information"=w329, "Error"=w336) -> ()  [unwired: 9 in, 1 out]
    }
  }
  n168 = Merge Errors(w18, w21) -> (w17:errorcluster)
  n169 = call "Close Module.vi"("error in"=w17, "Module Admin in"=w12) -> ("error out"=w19:errorcluster, "External Launch"=w5:bool, "Module Admin out"=w6:refnum<class "Delacor_lib_QMH_Module Admin.lvclass">)  [unwired: 7 in]
  n170 = Unregister For Events(event registration refnum=w11, error in=w19) -> (error out=w16:errorcluster)
  n171 = call "Module Name--constant.vi"() -> ("Module Name"=w3:string)  [unwired: 11 in]
  n172 = case "External Launch?" shown="True" w5 {
    tunnel: w16 -> [_ w337]
    frame False {
    }
    frame True {
      n173 = case shown="No Error" w337 {
        frame No Error {
          n174 = invoke class="VI" method="FP.Close"() -> ()  [unwired: 3 in, 3 out]
        }
        frame Error {
          n175 = invoke class="VI" method="FP.Open"("Activate"=TRUE ("Activate?")) -> ()  [unwired: 4 in, 5 out]
        }
      }
    }
  }
  n176 = local write "Module Admin"(w6) -> ()
  n177 = Format Into String(format string="Module %s stopped.", w3) -> (resulting string=w1:string)  [unwired: 2 in, 1 out]
  n178 = call <vilib>:"INFO.vi"("Message"=w1, "error in"=w16) -> ("error out"=→"error out":errorcluster)  [unwired: 9 in]
